vi "Post Message and Send Message to Non-Exist Module.vi"() -> ()   [LabVIEW 2014]
uses:
  user.lib/_NEVSTOP/JKI State Machine++/JKI State Machine++.lvlib
panel:
  out "error out 2":errorcluster
  out "error out":errorcluster
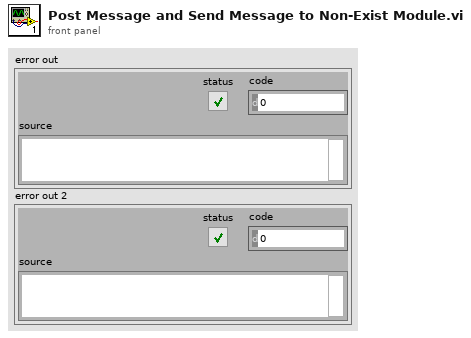
[diagram p1: front panel]
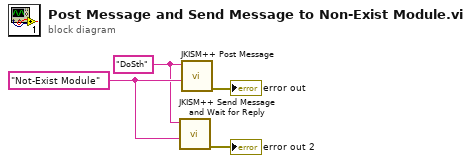
[diagram p0: block diagram]
diagram:
  w3 = "DoSth" ("States")
  w4 = "Not-Exist Module" ("Dest Module")
  n1 = call "JKISM++ Send Message and Wait for Reply.vi"("Target Module"=w4, "State"=w3) -> ("error out"=→"error out 2":errorcluster)  [unwired: 8 in, 1 out]
  n2 = call "JKISM++ Post Message.vi"("Target Module"=w4, "State"=w3) -> ("error out"=→"error out":errorcluster)  [unwired: 9 in]
